vi "Init.Mathematica.vi"(1 "Name":string) -> (0 "reference":refnum<k24>)   [LabVIEW 2014]
uses:
  D:/Desktop/app/LabVIEW/Wolfram.NETLink.dll
  Wolfram.NETLink.dll
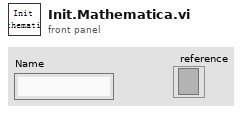
[diagram p1: front panel]
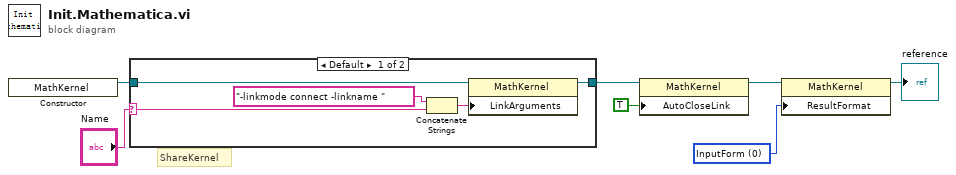
[diagram p0: block diagram]
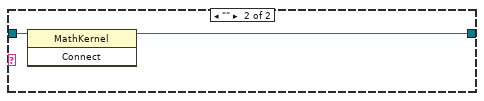
[diagram p2: hidden frame]
diagram:
  w7 = 0 items=["InputForm", "OutputForm", "StandardForm", "TraditionalForm", "MathML", "Expr"] ("ResultFormat")
  # "ShareKernel"
  n1 = constructor class="MathKernel"() -> (reference out=w3:refnum<k24>)  [unwired: 3 in, 2 out]
  n2 = case shown="Default" "Name" {
    selector: "Name" -> [w8 _]
    tunnel: w3 -> [w12 w14]
    tunnel: [w9 w13] -> w2
    frame Default {
      n3 = Concatenate Strings("-linkmode connect -linkname " ("string"), w8) -> (w10:string)
      n4 = property class="MathKernel"(reference=w12, "LinkArguments"=w10) -> (reference out=w9:refnum<k24>)  [unwired: 1 in, 1 out]
    }
    frame "" {
      n5 = invoke class="MathKernel" method="Connect"(reference=w14) -> (reference out=w13:refnum<k24>)  [unwired: 2 in, 2 out]
    }
  }
  n6 = property class="MathKernel"(reference=w2, "AutoCloseLink"=TRUE) -> (reference out=w6:refnum<k24>)  [unwired: 1 in, 1 out]
  n7 = property class="MathKernel"(reference=w6, "ResultFormat"=w7) -> (reference out=→"reference":refnum<k24>)  [unwired: 1 in, 1 out]
